vi "Read_File_No_Error.vi"(0 "Filename":path, 1 "number of characters (all:-1)":i32=-1, 3 "pos offset (bytes:0)":i32) -> (5 "error out":errorcluster, 6 "Error?":bool, 7 "Filename Out":path, 8 "string":string, 9 "EOF?":bool, 10 "mark after read (chars.)":i32)   [LabVIEW 2010]
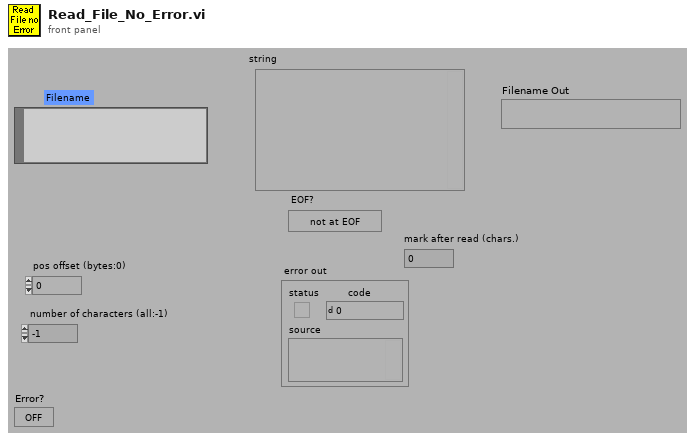
[diagram p1: front panel]
types:
  T1 = enum16{"read/write", "read-only", "write-only", "write-only (truncate)"}
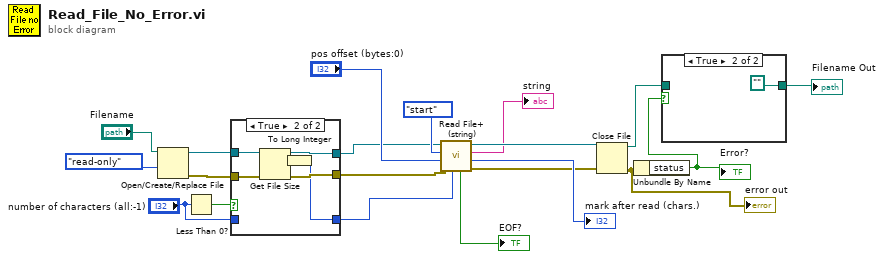
[diagram p0: block diagram]
diagram:
  n1 = Open/Create/Replace File(file path (use dialog)="Filename", access (0:read/write)=T1."read-only" ("open mode (0)")) -> (refnum out=w2:refnum<file>, error out=w1:errorcluster)  [unwired: 1 in, 4 out]
  n2 = Less Than 0?(x="number of characters (all:-1)") -> (x < 0?=w13:bool)
  n3 = case shown="True" w13 {
    tunnel: w2 -> [w23 w29]
    tunnel: w1 -> [w22 w28]
    tunnel: [w22 w27] -> w12
    tunnel: [w23 w26] -> w11
    tunnel: [w21 w25] -> w10
    tunnel: "number of characters (all:-1)" -> [w21 _]
    frame False {
    }
    frame True {
      n4 = Get File Size(file=w29, error in=w28) -> (refnum out=w26:refnum<file>, size (in bytes)=w24:i64, 0:w27:errorcluster)
      n5 = To Long Integer(number=w24) -> (32bit integer=w25:i32)
    }
  }
  n6 = call <vilib>:"Read File+ (string).vi"("count"=w10, "error in (no error)"=w12, "pos offset (bytes:0)"="pos offset (bytes:0)", "pos mode (rel. to current:2)"=enum16{"start", "end", "current"}."start", "refnum"=w11) -> ("error out"=w16:errorcluster, "mark after read (bytes)"=→"mark after read (chars.)":i32, "string"=→"string":string, "dup refnum"=w17:refnum<file>, "EOF?"=→"EOF?":bool)  [unwired: 2 out]
  n7 = Close File(refnum=w17, error in=w16) -> (path=w5:path, error out=w8:errorcluster)
  "error out" <- w8
  n8 = Unbundle By Name(w8) -> ("status"=w7:bool)
  "Error?" <- w7
  n9 = case shown="True" w7 {
    tunnel: [w30 path ""] -> w6
    tunnel: w5 -> [w30 _]
    frame False {
    }
    frame True {
    }
  }
  "Filename Out" <- w6
